vi "ExSpectSetSlitPosIN.vi"() -> ()   [LabVIEW 2010]
panel:
  in  "Slit Number":i16=1 min=1 max=4 step=1
  in  "Position":dbl format="%.2f"
  out "error out":errorcluster
  in  "error in (no error)":errorcluster
  # "ExSpectSetSlitPosIN.vi (InSpectrum)\nCamera and Spectrometer control of the InSpectrum.  This vi will open both the camera and spectrograph then set the current position of the selected slit."
  # "NOTES:\nDepending on the camera, a properly configured .INI file may be required in the WINDOWS folder for correct camera operation.\n\nA properly configured spectometer .ini must be present in the LabVIEW folder for spectrograph operation.\n\nConsult the Toolkit documentation for more information on how to configure these files."
  # "um"
  # "1 = Front Entrance\n 2 = Side Entrance\n 3 = Front Exit\n 4 = Side Exit"
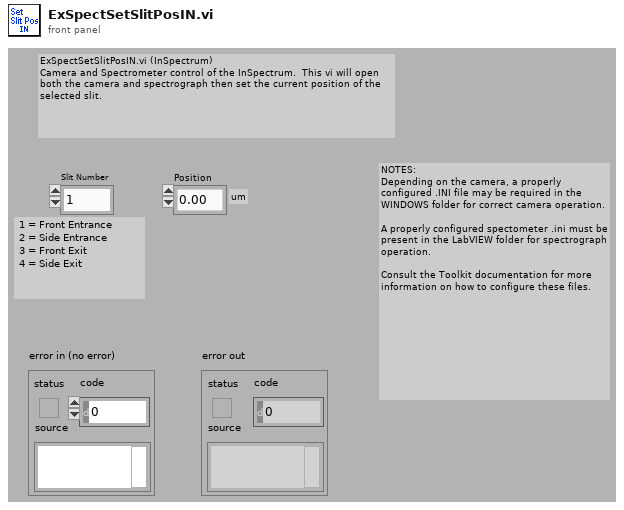
[diagram p1: front panel]
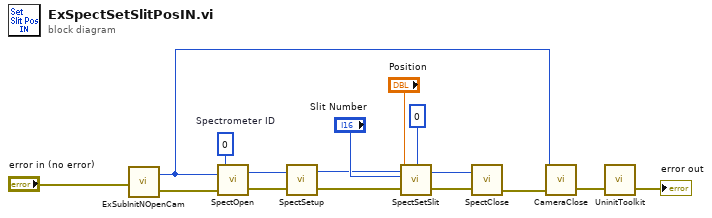
[diagram p0: block diagram]
diagram:
  w13 = u32 0  # Spectrometer ID
  n1 = call "ExSubInitNOpenCam.vi"("error in (no error)"="error in (no error)") -> ("Camera Handle"=w3:u32, "error out"=w12:errorcluster)
  n2 = call <userlib>:"SpectOpen.vi"("error in"=w12, "Camera Handle"=w3, "Spectrometer ID"=w13) -> ("error out"=w14:errorcluster, "Spectrometer Handle"=w15:u32)
  n3 = call <userlib>:"SpectSetup.vi"("error in"=w14, "Spectrometer Handle"=w15) -> ("error out"=w9:errorcluster, "Spectrometer Handle"=w10:u32)
  n4 = call <userlib>:"SpectSetSlit.vi"("Spectrometer Handle"=w10, "Slit Number"="Slit Number", "Position"="Position", "error in"=w9, "Speed"=0) -> ("Spectrometer Handle"=w4:u32, "error out"=w8:errorcluster)
  n5 = call <userlib>:"SpectClose.vi"("error in"=w8, "Spectrometer Handle"=w4) -> ("error out"=w7:errorcluster)
  n6 = call <userlib>:"CameraClose.vi"("error in"=w7, "Camera Handle"=w3) -> ("error out"=w6:errorcluster)
  n7 = call <userlib>:"UninitToolkit.vi"("error in"=w6) -> ("error out"=→"error out":errorcluster)
